vi "ManualOverrideOCU.vi"() -> ()   [LabVIEW 2011]
doc: "The Manual Override, first and foremost, allows the user to switch the boat from autonomous to override from the front panel. It's secondary function is to control the boat with keys. Currently the arrow keys connect to the sail, and the WASD keys connect to the rudder, as shown in the front panel labels. It is clearly illustrated how the keys change the value and then which values are sent to the global. You can easily change which keys do what by going to the back panel and changing the key tests.\n\nCreated by Eric Jones and Eric Schneider"
uses:
  2-Think/2 Typedefs/setpoints to boat.ctl
  2-Think/2 Typedefs/sail setpt.ctl
  2-Think/2 Typedefs/rudder angle.ctl
  0x2-OCU-Think Comm/0x2 Typedefs/manual override.ctl
  2-Think/2 Globals/2 Global.vi
panel:
  in  "OVERRIDE SAIL?":bool
  in  "OVERRIDE RUDDER?":bool
  in  "VI stop":bool
  out "Sent Rudder Angle":dbl(slide) scale=-30.0..30.0
  out "Sent Sail Value":dbl(slide) scale=0.0..1.0
  # "The Manual Override, first and foremost, allows the user to switch the boat from autonomous to override from the  front panel. It's secondary function is to control the boat with keys. Currently the arrow keys connect to the sail, and the ASDFG keys connect to the rudder, as shown in the front panel labels. It is clearly illustrated how the keys change the value and then which values are sent to the global. You can easily change which keys do what by going to the back panel and changing the key tests.\n\nToDo:\nPossibly implement a \"smart sails\" option that would allow the controller to only need to control the rudder and sails would be controlled by the boat based on heading, rudder angle, and apparent wind."
  # "SENT VALUES"
  # "SAIL CONTROL"
  # "Full Out = RIGHT"
  # "OUT = 1"
  # "Out = UP"
  # "In = DOWN"
  # "Full In = LEFT"
  # "IN = 0"
  # "RUDDER CONTROL"
  # "Full \nStarboard"
  # "Full \nPort"
  # "<--"
  # "Straight"
  # "-->"
  # "A"
  # "F"
  # "G"
  # "PORT = -30"
  # "STARB = 30"
  # "S"
  # "D"
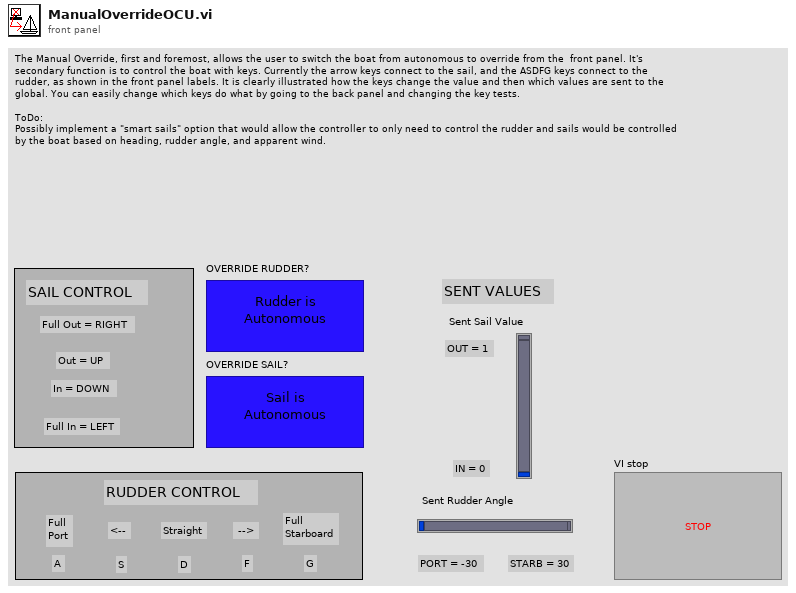
[diagram p1: front panel]
types:
  T1 = typedef "setpoints to boat.ctl" = cluster{"Sail Position":T2, "Rudder Angle":T3}
  T2 = typedef "sail setpt.ctl" = dbl
  T3 = typedef "rudder angle.ctl" = dbl
  T4 = typedef "manual override.ctl" = cluster{"Override Active Rudder":bool, "Setpoints":T1, "Override Active Sail":bool}
  T5 = typedef "eventvkey.ctl" = enum16{"ASCII", "Enter", "Return", "Shift", "Ctrl", "Alt", "Cmd", "Opt", "Caps", "NumLock", "Clear", "Break", "Up", "Down", "Left", "Right", "Insert", "Delete", "Home", "End", "PageUp", "PageDown", "Escape", "Help", "Pause", "ScrollLock", "F1", "F2", "F3", "F4", "F5", "F6", "F7", "F8", "F9", "F10", "F11", "F12", "F13", "F14", "F15", "F16", "F17", "F18", "F19", "F20", "F21", "F22", "F23", "F24", "Play", "VolumeUp", "VolumeDown", "Mute", "Two Byte Char"}
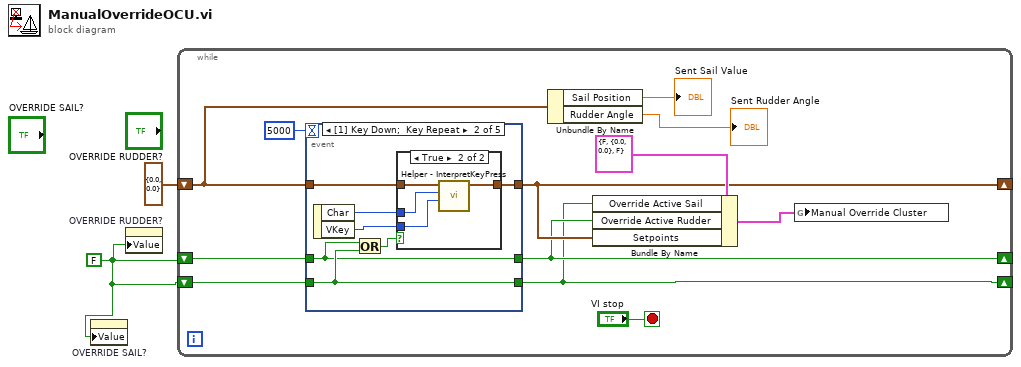
[diagram p0: block diagram]
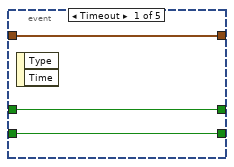
[diagram p2: hidden frame]
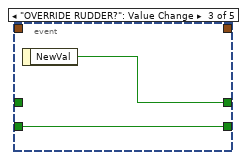
[diagram p4: hidden frame]
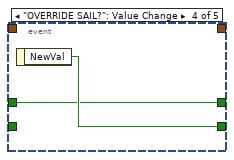
[diagram p5: hidden frame]
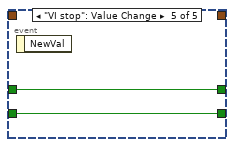
[diagram p6: hidden frame]
diagram:
  w1 = FALSE ("OVERRIDE?")
  n1 = property on="OVERRIDE SAIL?" class="Bool (strict)"("Value"=w1) -> ()  [unwired: 2 in, 2 out]
  n2 = property on="OVERRIDE RUDDER?" class="Bool (strict)"("Value"=w1) -> ()  [unwired: 2 in, 2 out]
  n3 = while {
    shift-right: [w8] -> _
    shift-left: T1 {"Sail Position"=0.0, "Rudder Angle"=0.0} -> [w6]
    shift-right: [w7] -> _
    shift-left: w1 -> [w9]
    shift-right: [w4] -> _
    shift-left: w1 -> [w5]
    stop <- "VI stop" stop-if-true
    n4 = event shown="[1] Key Down;  Key Repeat" {
      selector: _ -> [_ _ _ _ _]
      dyn-events: _ -> [_ _ _ _ _]
      timeout: 5000 -> [_ _ _ _ _]
      tunnel: w6 -> [w17 w24 _ _ _]
      tunnel: [w17 w23 _ _ _] -> w8
      tunnel: w9 -> [w16 w19 _ w32 w35]
      tunnel: [w16 w19 w31 w32 w35] -> w7
      tunnel: w5 -> [w15 w20 w30 _ w34]
      tunnel: [w15 w20 w30 w33 w34] -> w4
      event Timeout {
        n5 = event-data() -> ()  [unwired: 1 in, 2 out]
      }
      event Key Down; Key Repeat {
        n6 = event-data() -> ("Char"=w22:i16, "VKey"=w21:T5)  [unwired: 1 in]
        n7 = Or(x=w19, y=w20) -> (x .or. y?=w18:bool)
        n8 = case shown="True" w18 {
          tunnel: w24 -> [w25 w29]
          tunnel: [w25 w28] -> w23
          tunnel: w22 -> [_ w27]
          tunnel: w21 -> [_ w26]
          frame False {
          }
          frame True {
            n9 = call "Helper - InterpretKeyPress.vi"("VKey"=w26, "Char"=w27, "Command In"=w29) -> ("Command Out"=w28:T1)  [unwired: 8 in]
          }
        }
      }
      event "OVERRIDE RUDDER?": Value Change {
        n10 = event-data() -> ("NewVal"=w31:bool)  [unwired: 1 in]
      }
      event "OVERRIDE SAIL?": Value Change {
        n11 = event-data() -> ("NewVal"=w33:bool)  [unwired: 1 in]
      }
      event "VI stop": Value Change {
        n12 = event-data() -> ()  [unwired: 1 in, 1 out]
      }
    }
    n13 = Unbundle By Name(w6) -> ("Sail Position"=→"Sent Sail Value":T2, "Rudder Angle"=→"Sent Rudder Angle":T3)
    n14 = Bundle By Name(cluster=T4 {"Override Active Rudder"=FALSE, "Setpoints"={"Sail Position"=0.0, "Rudder Angle"=0.0}, "Override Active Sail"=FALSE}, "Override Active Sail"=w4, "Override Active Rudder"=w7, "Setpoints"=w8) -> (w13:T4)
    n15 = global write "2 Global.vi" "Manual Override Cluster"(w13) -> ()
  }
